vi "Init Module.vi"(8 "error in":errorcluster, 10 "Close Master Reference (F)":bool, 11 "Cloneable Module Admin in":refnum<class "Delacor_lib_QMH_Cloneable Module Admin.lvclass">) -> (0 "error out":errorcluster, 2 "Power Supply Request Events":T1, 3 "Cloneable Module Admin out":refnum<class "Delacor_lib_QMH_Cloneable Module Admin.lvclass">)   [LabVIEW 2025, in "Power Supply.lvlib"]
doc: "Initialize the module by creating Broadcast Events, Request Events, and synchronization rendezvous. Also, since this is a cloneable module, add it to the cloneable registry and update the Module Admin class.\n\nSee the block diagram for an explanation of the 'Close Master Reference' parameter.\n_____\nBased on DQMH Dev Tools: Project Template 7.1.2.1547."
uses:
  Power Supply.lvlib
  <vilib>/Delacor/Delacor QMH/Libraries/Cloneable Module Admin_class/Delacor_lib_QMH_Cloneable Module Admin.lvclass
  C:/Program Files/National Instruments/LabVIEW 2025/vi.lib/Delacor/Delacor QMH/Libraries/Module Admin_class/Delacor_lib_QMH_Module Admin.lvclass
  Request Events--cluster.ctl
  Stop Argument--cluster.ctl
  Show Panel Argument--cluster.ctl
  Hide Panel Argument--cluster.ctl
  Show Diagram Argument--cluster.ctl
  Get Module Execution Status Argument--cluster.ctl
  select child Argument--cluster.ctl
  Classes/hardware-selection.ctl
  select child (Reply Payload)--cluster.ctl
  read config Argument--cluster.ctl
  read config (Reply Payload)--cluster.ctl
  init device Argument--cluster.ctl
  init device (Reply Payload)--cluster.ctl
  close Argument--cluster.ctl
  close (Reply Payload)--cluster.ctl
  output Argument--cluster.ctl
  output (Reply Payload)--cluster.ctl
  set voltage Argument--cluster.ctl
  set voltage (Reply Payload)--cluster.ctl
  set current Argument--cluster.ctl
  set current (Reply Payload)--cluster.ctl
  read current Argument--cluster.ctl
  read current (Reply Payload)--cluster.ctl
  Controls/Numeric Current.ctl
  read voltage Argument--cluster.ctl
  read voltage (Reply Payload)--cluster.ctl
  Controls/Numeric Voltage.ctl
  read state Argument--cluster.ctl
  read state (Reply Payload)--cluster.ctl
  set all outputs Argument--cluster.ctl
  set all outputs (Reply Payload)--cluster.ctl
  <vilib>/Delacor/Delacor QMH/Libraries/Module Admin_class/Delacor_lib_QMH_Module Admin.lvclass/Delacor_lib_QMH_Module Admin.ctl
  <vilib>/Delacor/Delacor QMH/Libraries/Cloneable Module Admin_class/Delacor_lib_QMH_Cloneable Module Admin.lvclass/Delacor_lib_QMH_Cloneable Module Admin.ctl
  <vilib>/Delacor/Delacor QMH/Libraries/Module Admin_class/Delacor_lib_QMH_Get External Launch.vi
  <vilib>/Delacor/Delacor QMH/Libraries/Cloneable Module Admin_class/Delacor_lib_QMH_Get Module ID.vi
  <vilib>/Delacor/Delacor QMH/Libraries/Cloneable Module Admin_class/Delacor_lib_QMH_Set Close Master Reference.vi
  <vilib>/Delacor/Delacor QMH/Libraries/Cloneable Module Admin_class/Delacor_lib_QMH_Set First.vi
  Clone Registration/Clone Registration.lvlib
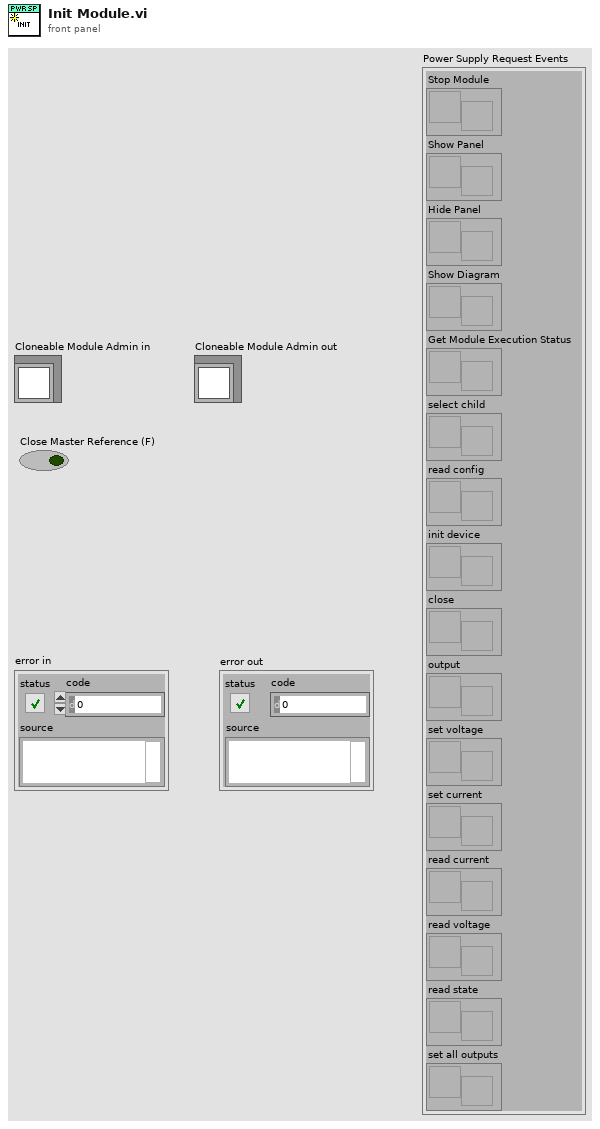
[diagram p1: front panel]
types:
  T1 = typedef "Power Supply.lvlib/Request Events--cluster.ctl" = cluster{"Stop Module":refnum<user-event>, "Show Panel":refnum<user-event>, "Hide Panel":refnum<user-event>, "Show Diagram":refnum<user-event>, "Get Module Execution Status":refnum<user-event>, "select child":refnum<user-event>, "read config":refnum<user-event>, "init device":refnum<user-event>, "close":refnum<user-event>, "output":refnum<user-event>, "set voltage":refnum<user-event>, "set current":refnum<user-event>, "read current":refnum<user-event>, "read voltage":refnum<user-event>, "read state":refnum<user-event>, "set all outputs":refnum<user-event>}
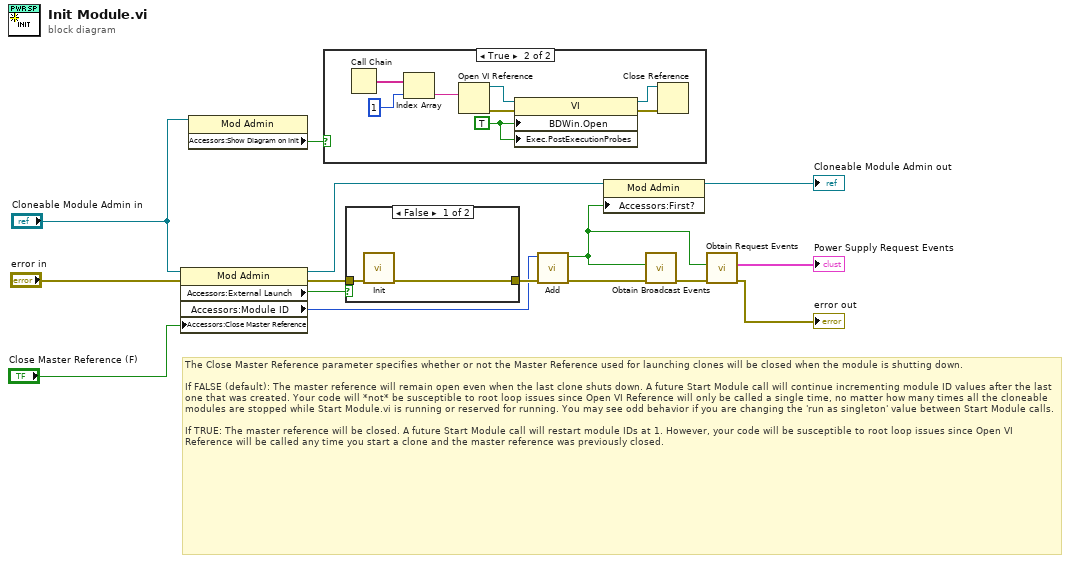
[diagram p0: block diagram]
diagram:
  # "The Close Master Reference parameter specifies whether or not the Master Reference used for launching clones will be closed when the module is shutting down. \n\nIf FALSE (default): The master reference will remain open even when the last clone shuts down. A future Start Module call will continue incrementing module ID values after the last one that was created. Your code will *not* be susceptible to root loop issues since Open VI Reference will only be called a single time, no matter how many times all the cloneable modules are stopped while Start Module.vi is running or reserved for running. You may see odd behavior if you are changing the 'run as singleton' value between Start Module calls.\n\nIf TRUE: The master reference will be closed. A future Start Module call will restart module IDs at 1. However, your code will be susceptible to root loop issues since Open VI Reference will be called any time you start a clone and the master reference was previously closed."
  n1 = property class="Mod Admin"(reference="Cloneable Module Admin in", error in="error in", "Accessors:Close Master Reference"="Close Master Reference (F)") -> (reference out=w9:refnum<class "Delacor_lib_QMH_Cloneable Module Admin.lvclass">, error out=w5:errorcluster, "Accessors:External Launch"=w8:bool, "Accessors:Module ID"=w4:i32)
  n2 = property class="Mod Admin"(reference="Cloneable Module Admin in") -> ("Accessors:Show Diagram on Init"=w2:bool)  [unwired: 1 in, 2 out]
  n3 = case shown="True" w2 {
    frame False {
    }
    frame True {
      w19 = TRUE ("Block Diagram Window:Open")
      n4 = Call Chain() -> (call chain=w23:string[])
      n5 = Index Array(array=w23, index=1) -> (element=w16:string)
      n6 = Open VI Reference(vi path=w16) -> (vi reference=w20:refnum<vi>, error out=w21:errorcluster)  [unwired: 5 in]
      n7 = property class="VI"(reference=w20, error in=w21, "BDWin.Open"=w19, "Exec.PostExecutionProbes"=w19) -> (reference out=w17:refnum<vi>, error out=w18:errorcluster)
      n8 = Close Reference(reference=w17, error in (no error)=w18) -> ()  [unwired: 1 out]
    }
  }
  n9 = case "External Launch?" shown="False" w8 {
    tunnel: [w25 w26] -> w14
    tunnel: w5 -> [w24 w26]
    frame False {
      n10 = call "Init.vi"("error in"=w24) -> ("error out"=w25:errorcluster)  [unwired: 7 in, 3 out]
    }
    frame True {
      # "Init of Clone's registration\nhappened at Start Module.vi"
    }
  }
  n11 = call "Add.vi"("error in"=w14, "Module ID"=w4) -> ("error out"=w15:errorcluster, "First?"=w10:bool)  [unwired: 7 in, 1 out]
  n12 = property class="Mod Admin"(reference=w9, "Accessors:First?"=w10) -> (reference out=→"Cloneable Module Admin out":refnum<class "Delacor_lib_QMH_Cloneable Module Admin.lvclass">)  [unwired: 1 in, 1 out]
  n13 = call "Obtain Broadcast Events.vi"("error in"=w15, "Create New? (F)"=w10) -> ("error out"=w13:errorcluster)  [unwired: 8 in, 1 out]
  n14 = call "Obtain Request Events.vi"("error in"=w13, "Create New? (F)"=w10) -> ("error out"=→"error out":errorcluster, "Power Supply Request Events"=→"Power Supply Request Events":T1)  [unwired: 8 in]
